vi "Time to Match Brian Sheridan.vi"() -> ()   [LabVIEW 2014]
panel:
  out "Time to Match":dbl format="%#.3f"
  out "# of iterations":i32 format="%#.0f"
  out "Current Number":i32 format="%#.0f"
  in  "Number to Match":i32 min=0 max=1000 step=1 format="%#.0f"
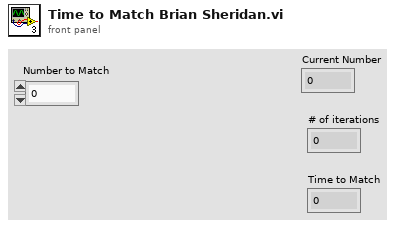
[diagram p1: front panel]
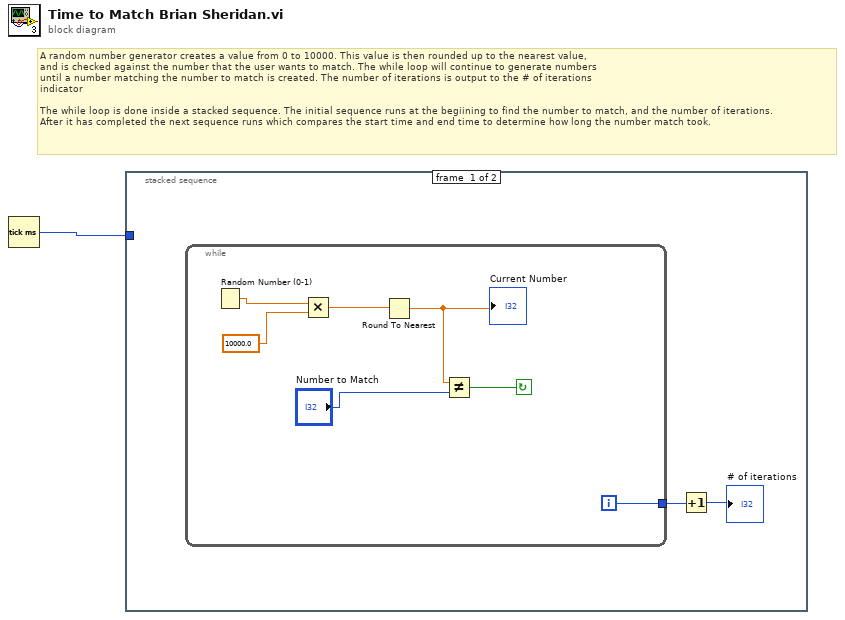
[diagram p0: block diagram]
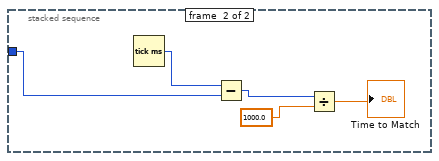
[diagram p2: hidden frame]
diagram:
  # "A random number generator creates a value from 0 to 10000. This value is then rounded up to the nearest value,\nand is checked against the number that the user wants to match. The while loop will continue to generate numbers \nuntil a number matching the number to match is created. The number of iterations is output to the # of iterations \nindicator\n\nThe while loop is done inside a stacked sequence. The initial sequence runs at the begiining to find the number to match, and the number of iterations.\nAfter it has completed the next sequence runs which compares the start time and end time to determine how long the number match took."
  n1 = Tick Count (ms)() -> (millisecond timer value=w1:u32)
  n2 = stacked-sequence {
    tunnel: w1 -> [_ w12]
    frame #0 {
      n3 = while {
        tunnel: [w4] -> w2
        i -> [w4]
        stop <- w7 continue-if-true
        n4 = Random Number (0-1)() -> (number: 0 to 1=w10:dbl)
        n5 = Multiply(x=w10, y=10000.0) -> (x*y=w8:dbl)
        n6 = Round To Nearest(number=w8) -> (nearest integer value=w5:dbl)
        "Current Number" <- w5
        n7 = Not Equal?(x=w5, y="Number to Match") -> (x != y?=w7:bool)
      }
      n8 = Increment(x=w2) -> (x+1=→"# of iterations":i32)
    }
    frame #1 {
      n9 = Tick Count (ms)() -> (millisecond timer value=w11:u32)
      n10 = Subtract(x=w11, y=w12) -> (x-y=w13:u32)
      n11 = Divide(x=w13, y=1000.0) -> (x/y=→"Time to Match":dbl)
    }
  }
